vi "test_Spectral transform.vi"() -> ()   [LabVIEW 2014]
uses:
  Melody Extraction.lvlib
panel:
  out "Intensity Graph":dbl[][](graph)
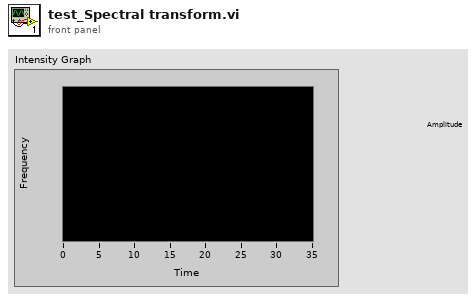
[diagram p1: front panel]
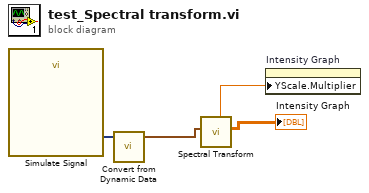
[diagram p0: block diagram]
diagram:
  n1 = call "Simulate Signal"() -> ("Square"=w4:dynamicdata)  [unwired: 14 in, 1 out]
  n2 = call "Convert from Dynamic Data"("Dynamic Data Type"=w4) -> ("Waveform"=w1:waveform(dbl))  [unwired: 3 in]
  n3 = call "Spectral Transform.vi"("Input Waveform"=w1) -> ("STFT"=→"Intensity Graph":dbl[][], "Frequency Axis Scale Factor"=w2:dbl)  [unwired: 9 in]
  n4 = property on="Intensity Graph" class="IntGraph (strict)"("YScale.Multiplier"=w2) -> ()  [unwired: 2 in, 2 out]
